vi "titration_point.vi"(6 "Small HCl incriment":dbl, 7 "Dosimat In":T1={"Dosimat Port in"="COM1", "Error in"={"status"=FALSE, "code"=0, "source"=""}}) -> (0 "EMF 1":dbl, 1 "Total HCl Volume":dbl, 2 "Cell Temp":dbl, 3 "Dosimat Out":T2={"Dosimat Port out"="COM1", "Error out"={"status"=FALSE, "code"=0, "source"=""}}, 4 "EMF 2":dbl)   [LabVIEW 2010]
uses:
  HCl_volume_global.vi
panel:
  # "This is one of the meaty routines that actually performs the titration… \nafter the initial dose of acid gets added, this vi adds small increments of acid a\nnd takes measurements from the pH and temperature probes. \nIn new routine, we will skip reading gas flow (just record whether it was on High or Low)… \nThis sends data to an XY plot that is pretty klugy. \nImportant inputs are small HCl increments (set by user) and number of titration points (calculated in 2 different vis).\n\nStep 0 of the sequence structure will need to be modified with Dosimat876 routines. \n\nEMF filter is a bool to decide whether to report back the pH voltage in addition to the tmep\n\nThis would be another candidate for some good error checking"
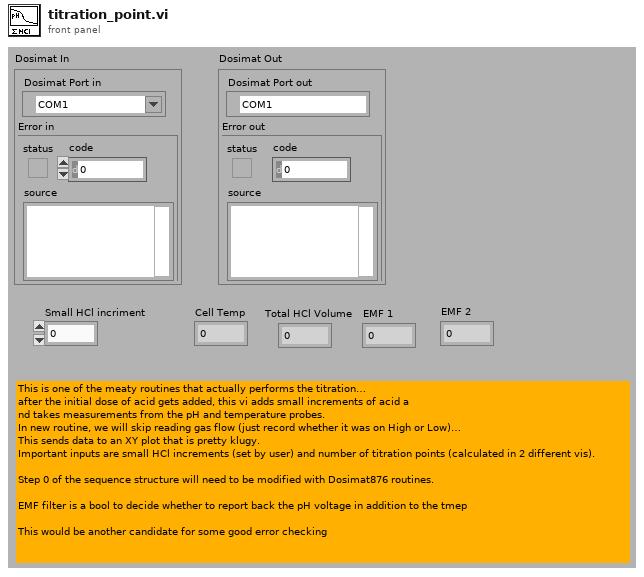
[diagram p1: front panel]
types:
  T1 = cluster{"Dosimat Port in":refnum<visa-resource-name>, "Error in":errorcluster}
  T2 = cluster{"Dosimat Port out":refnum<visa-resource-name>, "Error out":errorcluster}
  T3 = cluster{"Dosimat Port Out":refnum<visa-resource-name>, "error out":errorcluster}
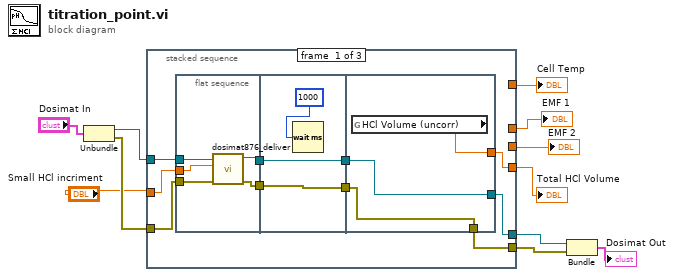
[diagram p0: block diagram]
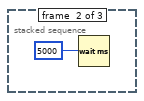
[diagram p2: hidden frame]
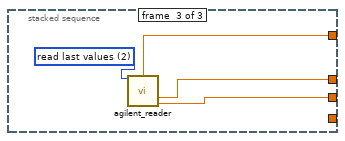
[diagram p3: hidden frame]
diagram:
  n1 = Unbundle("Dosimat In") -> ("Dosimat Port in"=w10:refnum<visa-resource-name>, "Error in"=w9:errorcluster)
  n2 = stacked-sequence {
    tunnel: w9 -> [w19 _ _]
    tunnel: [w16 _ _] -> w6
    tunnel: [w15 _ _] -> w7
    tunnel: w10 -> [w14 _ _]
    tunnel: "Small HCl incriment" -> [w13 _ _]
    tunnel: [_ _ w36] -> w4
    tunnel: [_ _ w35] -> w3
    tunnel: [_ _ w34] -> w2
    tunnel: [w12 _ _] -> w1
    frame #0 {
      # "Error Links"
      n3 = flat-sequence {
        tunnel: [w26] -> w21
        tunnel: w14 -> [w25]
        tunnel: w13 -> [w23]
        tunnel: w19 -> [w24]
        tunnel: [w22] -> w17
        tunnel: w21 -> [w29]
        tunnel: [w29] -> w20
        tunnel: [w27] -> w18
        tunnel: w17 -> [w27]
        tunnel: w20 -> [w32]
        tunnel: w18 -> [w31]
        tunnel: [w31] -> w16
        tunnel: [w32] -> w15
        tunnel: [w30] -> w12
        frame #0 {
          n4 = call "dosimat876_deliver.vi"("error in"=w24, "Volume"=w23, "Dosimat Port In"=w25) -> ("error out"=w22:errorcluster, "Dosimat Port Out"=w26:refnum<visa-resource-name>)  [unwired: 1 in, 2 out]
        }
        frame #1 {
          n5 = Wait (ms)(milliseconds to wait=1000) -> ()  [unwired: 1 out]
        }
        frame #2 {
          n6 = global read "HCl_volume_global.vi" "HCl Volume (uncorr)"() -> (w30:dbl)
        }
      }
    }
    frame #1 {
      n7 = Wait (ms)(milliseconds to wait=5000) -> ()  [unwired: 1 out]
    }
    frame #2 {
      w37 = u8 2 items=["read new values"=1, "read last values "=2] ("Action")
      n8 = call "agilent_reader.vi"("Action"=w37) -> ("Cell Temp"=w36:dbl, "Voltage 1"=w35:dbl, "Voltage 2"=w34:dbl)  [unwired: 3 in, 9 out]
    }
  }
  "EMF 1" <- w3
  "Total HCl Volume" <- w1
  "Cell Temp" <- w4
  "EMF 2" <- w2
  n9 = Bundle("Dosimat Port Out"=w7, "error out"=w6) -> (→"Dosimat Out":T3)  [unwired: 1 in]
